vi "Send.vi"(9 "Nest Alias":string, 10 "Nest Actor":refnum<class "Actor.lvclass">) -> (3 "Actor Create Msg Strategy out":refnum<class "Actor Create Msg Strategy.lvclass">)   [LabVIEW 2021, in "Actor Create.lvlib" / "Actor Create Msg Strategy.lvclass"]
uses:
  Actor Create Msg Strategy.lvclass
  LVCAM/Actor/Actor.lvclass
  Actor Create Msg Strategy.lvclass/Actor Create Msg Strategy.ctl
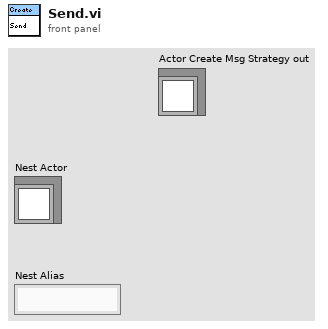
[diagram p1: front panel]
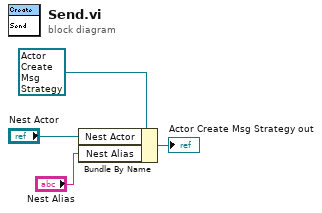
[diagram p0: block diagram]
diagram:
  n1 = Bundle By Name(cluster=refnum<class "Actor Create Msg Strategy.lvclass"> refnum ("Create Msg in"), "Nest Actor"="Nest Actor", "Nest Alias"="Nest Alias") -> (→"Actor Create Msg Strategy out":refnum<class "Actor Create Msg Strategy.lvclass">)
